vi "Alazar_ChannelConfig - ATS-SDK.vi"(4 "error in (no error)":errorcluster, 5 "V scale":T1 {"Coupling" items=["DC 1 MOhm", "AC 1 MOhm", "DC 50 Ohm", "AC 50 OHM"]; "Offset" format="%.2f"}, 6 "Channel":u8(ring)=1 items=["A"=1, "B"=2, "C"=4, "D"=8], 7 "Handle in":u32) -> (0 "error out":errorcluster, 1 "Return":u32, 3 "Handle_Out":u32)   [LabVIEW 2022 SP3]
panel:
  in  "Range":u32(ring)=33 items=["20 mV"=1, "40 mV"=2, "50 mV"=3, "80 mV"=4, "100 mV"=5, "200 mV"=6, "400 mV"=7, "500 mV"=8, "800 mV"=9, "1 V"=10, "1.25 V"=33, "2 V"=11, "4 V"=12, "5 V"=13, "8 V"=14, "10 V"=15, "20 V"=16]
  # "Need these values for a lookup. Integer value list needs to be pulled out."
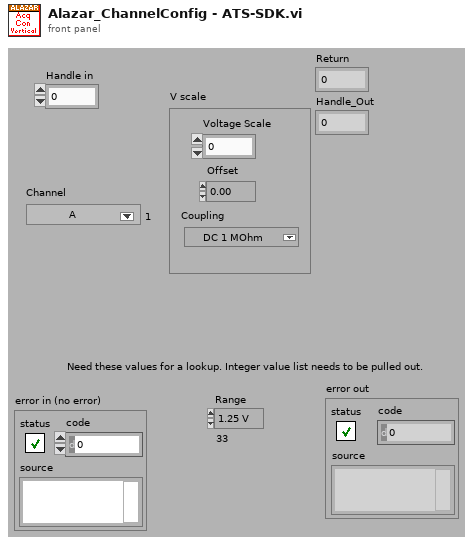
[diagram p1: front panel]
types:
  T1 = cluster{"Voltage Scale":dbl, "Offset":dbl, "Coupling":u16}
  T2 = typedef "LVStringsAndValuesArrayTypeDef_U32.ctl" = cluster{"String":string, "Value":u32}[]
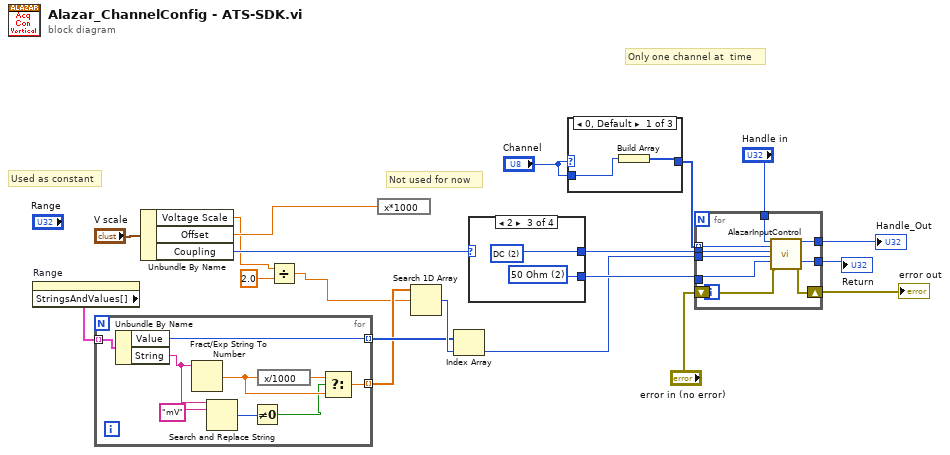
[diagram p0: block diagram]
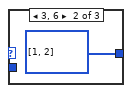
[diagram p2: hidden frame]
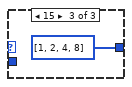
[diagram p3: hidden frame]
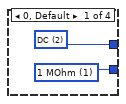
[diagram p4: hidden frame]
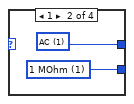
[diagram p5: hidden frame]
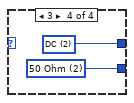
[diagram p6: hidden frame]
diagram:
  # "Only one channel at  time"
  # "Used as constant"
  # "Not used for now"
  n1 = property on="Range" class="Ring (strict)"() -> ("StringsAndValues[]"=w10:T2)  [unwired: 2 in, 2 out]
  n2 = for {
    tunnel: w10 -> [w29] mode=indexing
    tunnel: [w28] -> w9 mode=indexing
    tunnel: [w21] -> w6 mode=indexing
    n3 = Unbundle By Name(w29) -> ("Value"=w28:u32, "String"=w23:string)
    n4 = Fract/Exp String To Number(string=w23) -> (number=w26:dbl)  [unwired: 3 in, 1 out]
    n5 = Search and Replace String(input string=w23, search string="mV" ("format string")) -> (number of replacements=w24:i32)  [unwired: 6 in, 3 out]
    n6 = Not Equal To 0?(x=w24) -> (x != 0?=w22:bool)
    n7 = expression code="x/1000"(w26) -> (w27:dbl)
    n8 = Select(t=w27, s=w22, f=w26) -> (s? t:f=w21:dbl)
  }
  n9 = Unbundle By Name("V scale") -> ("Voltage Scale"=w5:dbl, "Offset"=w18:dbl, "Coupling"=w19:u16)
  n10 = Divide(x=w5, y=2.0) -> (x/y=w3:dbl)
  n11 = expression code="x*1000"(w18) -> ()  [unwired: 1 out]
  n12 = Search 1D Array(1D array=w6, element=w3) -> (index of element=w17:i32)  [unwired: 1 in]
  n13 = Index Array(array=w9, index=w17) -> (element=w11:u32)
  n14 = case shown="2" w19 {
    tunnel: [w31 w32 w35 w37] -> w14
    tunnel: [w30 w33 w34 w36] -> w13
    frame 0, Default {
      w30 = u32 1 items=["1 MOhm"=1, "50 Ohm"=2, ""=0] ("Impedance")
      w31 = u32 2 items=["AC"=1, "DC"=2] ("Coupling")
    }
    frame 1 {
      w32 = u32 1 items=["AC"=1, "DC"=2] ("Coupling")
      w33 = u32 1 items=["1 MOhm"=1, "50 Ohm"=2, ""=0] ("Impedance")
    }
    frame 2 {
      w34 = u32 2 items=["1 MOhm"=1, "50 Ohm"=2, ""=0] ("Impedance")
      w35 = u32 2 items=["AC"=1, "DC"=2] ("Coupling")
    }
    frame 3 {
      w36 = u32 2 items=["1 MOhm"=1, "50 Ohm"=2, ""=0] ("Impedance")
      w37 = u32 2 items=["AC"=1, "DC"=2] ("Coupling")
    }
  }
  n15 = case shown="0, Default" "Channel" {
    tunnel: [w38 w40 w41] -> w1
    tunnel: "Channel" -> [w39 _ _]
    frame 0, Default {
      n16 = Build Array(w39) -> (w38:u8[])
    }
    frame 3, 6 {
      w40 = u8[] [1, 2] items=["A"=1, "B"=2, "C"=4, "D"=8]
    }
    frame 15 {
      w41 = u8[] [1, 2, 4, 8] items=["A"=1, "B"=2, "C"=4, "D"=8]
    }
  }
  n17 = for {
    tunnel: [w50] -> w16
    tunnel: "Handle in" -> [w49]
    tunnel: w1 -> [w48] mode=indexing
    tunnel: w14 -> [w47]
    tunnel: w13 -> [w46]
    tunnel: [w45] -> w12
    tunnel: w11 -> [w44]
    shift-right: [w42] -> w7
    shift-left: "error in (no error)" -> [w43]
    n18 = call "AlazarInputControl.vi"("Handle"=w49, "Channel"=w48, "Coupling"=w47, "Range"=w44, "Impedance"=w46, "error in (no error)"=w43) -> ("Handle"=w50:u64, "Return Code"=w45:u32, "error out"=w42:errorcluster)  [unwired: 11 in]
  }
  "Return" <- w12
  "Handle_Out" <- w16
  "error out" <- w7
